vi "Drive Controller.vi"(8 "error in":errorcluster) -> ()   [LabVIEW 2020]
doc: "This VI executes continuously carrying out the current operation and responding to updates or new operation requests. It will often contain the timing or control code that is difficult to place directly in TeleOp. This VI generally opens all sensors and motors and isolates the rest of the robot code from knowing implementation details of how the operations are carried out."
uses:
  <vilib>/Rock Robotics/WPI/ThirdParty/REV Robotics/REVLib/Typedef/Spark MAX Control Type.ctl
  Drive Setpoints.ctl
  Drive Operations.ctl
  swerve/Type Definitions/Data/Robot Velocities.ctl
  <vilib>/Platform/TimedLoop/XDataNode/timing_clust.ctl
  <vilib>/Platform/TimedLoop/XDataNode/nitl_modes.ctl
  <vilib>/Platform/TimedLoop/XDataNode/wakeup.ctl
  <vilib>/Rock Robotics/WPI/ThirdParty/Phoenix-LabVIEW/Motor Controller/Controls/CTRE_Phoenix_MotorControl_ControlMode.ctl
  <vilib>/Rock Robotics/WPI/DriverStation/WPI_DriverStationRobotMode2.ctl
  9a6d1fe9-8481-493e-9338-0d478725c978.vi
  <vilib>/Analysis/_algsub.llb/Real Vector Norm.vi
  <vilib>/Analysis/coordinate.llb/2D Cartesian Coordinate Rotation (Scalar).vi
  Framework/Robot Global Data.vi
  <vilib>/Platform/TimedLoop/XDataNode/XDataNode.xnode
  <vilib>/Analysis/NI_AALPro.lvlib
  <vilib>/Platform/TimedLoop/XDataNode/XDNodeRunTimeDep.lvlib
panel:
  in  "Drive Controller Diagnostics":T1(tab)
  out "Swerve Visualizer":cluster{dbl[], dbl[]}[](graph)
  out "Pod Comparisons (Diff -> Setpoint - Actual)":T2
  out "Robot Pose":cluster{cluster{dbl, dbl}[]}[](graph)
  out "Robot Velocities (ft and deg)/s":cluster{"vx":dbl, "vy":dbl, "w":dbl}
  out "Robot Position (ft)":cluster{"x":dbl, "y":dbl, "theta":dbl}
  in  "Reset Pose":cluster{"vx":dbl, "vy":dbl, "w":dbl}
  in  "Reset?":bool
  out "Speed":dbl
  in  "Reserve Setpoints":T3
  in  "Reserve Control Mode":T4
  in  "Reserve Add Angle Offsets?":bool
  out "Auto Time Delta (ms)":u32(graph)
  out "(Calibration) Steering Angles":T3
  out "Current\nCmd":string
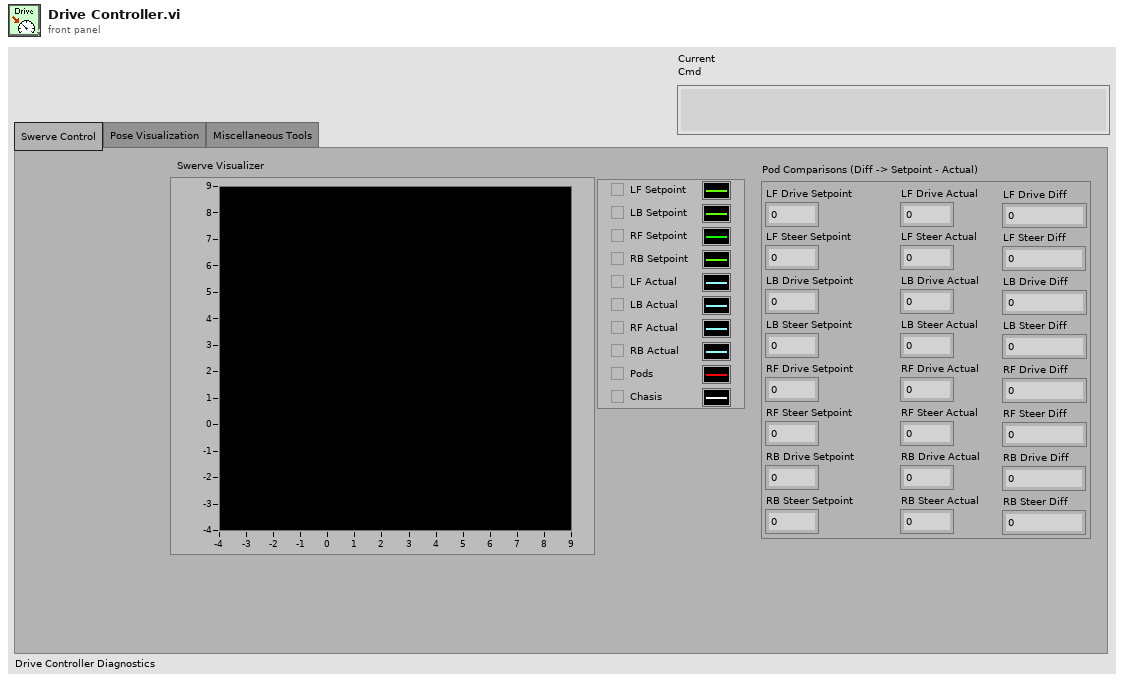
[diagram p1: front panel]
types:
  T1 = enum32{"Swerve Control", "Pose Visualization", "Miscellaneous Tools"}
  T2 = cluster{"LF Drive Setpoint":dbl, "LF Steer Setpoint":dbl, "LB Drive Setpoint":dbl, "LB Steer Setpoint":dbl, "RF Drive Setpoint":dbl, "RF Steer Setpoint":dbl, "RB Drive Setpoint":dbl, "RB Steer Setpoint":dbl, "LF Drive Actual":dbl, "LF Steer Actual":dbl, "LB Drive Actual":dbl, "LB Steer Actual":dbl, "RF Drive Actual":dbl, "RF Steer Actual":dbl, "RB Drive Actual":dbl, "RB Steer Actual":dbl, "LF Drive Diff":dbl, "LF Steer Diff":dbl, "LB Drive Diff":dbl, "LB Steer Diff":dbl, "RF Drive Diff":dbl, "RF Steer Diff":dbl, "RB Drive Diff":dbl, "RB Steer Diff":dbl}
  T3 = cluster{"Left Front":dbl, "Left Back":dbl, "Right Front":dbl, "Right Back":dbl}
  T4 = typedef "Spark MAX Control Type.ctl" = enum16{"Percent VBus", "Voltage", "Velocity", "Position", "Smart Motion", "Current", "Smart Velocity"}
  T5 = cluster{"Time (s)":dbl, "Command out":cluster{"Name":string, "vi reference":refnum<vi>, i32[], variant[]}}
  T6 = typedef "Drive Setpoints.ctl" = cluster{"Operation":T7, "Robot Velocities":T8, "Auto Data":cluster{"Auto Velocities":T8[], "Auto Positions":cluster{"x":dbl, "y":dbl, "th":dbl}[], "Auto Commands":cluster{dbl, "Command out":cluster{"Name":string, "vi reference":refnum<vi>, i32[], variant[]}}[], "Zero Velocity?":bool[]}, "Auto Engage Heading":bool}
  T7 = typedef "Drive Operations.ctl" = enum16{"Reserve", "Read Current", "Immediate", "Calibrate", "Auto", "Auto Engage", "Brake"}
  T8 = typedef "Robot Velocities.ctl" = cluster{"X Velocity":dbl, "Y Velocity":dbl, "Rotational \nVelocity":dbl}
  T9 = typedef "(NEO-NEO-ThroughBore-Pigeon2) Swerve.ctl" = cluster{"Drive Motors (NEO)":T10, "Steer Motors (NEO)":T10, "Pigeon2":T16, "Radii (ft)":T18}
  T10 = typedef "(NEO & NEO 550) 4 Motor Set.ctl" = cluster{"Left Front":T11, "Left Back":T11, "Right Front":T11, "Right Back":T11}
  T11 = typedef "WPI_MotorControlDeviceRef.ctl" = cluster{"DeviceStatus":errorcluster, "Type":T12, "PWM":cluster{"PWM Channel":T13, "DeadBand":T14}, "CAN":cluster{"Device Number":u8, "SetOutput VI Ref":variant, "GetOutput VI Ref":variant, "Enable VI Ref":variant, "Disable VI Ref":variant, "Data":variant}, "Invert":bool, "DIO PWM":cluster{"PWM \"Enable\" Channel":T13, "DIOChannel":T15, "PWM Rate":dbl}}
  T12 = typedef "WPI_MotorControlType.ctl" = enum16{"PWM", "CAN", "DIO PWM"}
  T13 = typedef "FPGA_DIOPWMChannel.ctl" = enum8{"PWM 0", "PWM 1", "PWM 2", "PWM 3", "PWM 4", "PWM 5", "PWM 6", "PWM 7", "PWM 8", "PWM 9", "PWM MXP 0", "PWM MXP 1", "PWM MXP 2", "PWM MXP 3", "PWM MXP 4", "PWM MXP 5", "PWM MXP 6", "PWM MXP 7", "PWM MXP 8", "PWM MXP 9", "Invalid"}
  T14 = typedef "WPI_PWMDeadband.ctl" = cluster{"Name":string, "maxPositivePwm":i32, "minPositivePwm":i32, "centerPwm":i32, "maxNegativePwm":i32, "minNegativePwm":i32, "angularRange":u16}
  T15 = typedef "FPGA_DIOChannel.ctl" = enum8{"DIO 0", "DIO 1", "DIO 2", "DIO 3", "DIO 4", "DIO 5", "DIO 6", "DIO 7", "DIO 8", "DIO 9", "DIO MXP 0", "DIO MXP 1", "DIO MXP 2", "DIO MXP 3", "DIO MXP 4", "DIO MXP 5", "DIO MXP 6", "DIO MXP 7", "DIO MXP 8", "DIO MXP 9", "DIO MXP 10", "DIO MXP 11", "DIO MXP 12", "DIO MXP 13", "DIO MXP 14", "DIO MXP 15", "SPI Port CS1", "SPI Port CS2", "SPI Port CS3", "SPI Port MISO", "SPI Port MOSI", "Invalid"}
  T16 = typedef "CTRE_PigeonIMU_DeviceRef.ctl" = cluster{"DeviceStatus":errorcluster, "Device Number":u8, "Type":T17, "Device ID":u32, "Handle":u64, "UsageFrame":u32, "Library Path":path}
  T17 = typedef "CTRE_PigeonIMU_ConnectionType.ctl" = u32
  T18 = typedef "Pod Positions.ctl" = cluster{"Left Front Position":dbl[], "Left Back Position":dbl[], "Right Front Position":dbl[], "Right Back Position":dbl[]}
  T19 = typedef "Command Status Info.ctl" = cluster{"Name":string, "Status":T20, "notifier out":T21}
  T20 = typedef "Completion Status.ctl" = enum16{"Successful", "Aborted", "Incomplete"}
  T21 = typedef "Completion Notifier.ctl" = refnum<notifier>
  T22 = cluster{"SubSystem Data":T6, cluster{"Start Time (ms)":u32, "Iterations":i32}, cluster{"Command Info":T19, "Description":string, "Default Command":T6, "queue out":refnum<queue>, "Subsystem Name":string}}
  T23 = cluster{"Auto Velocities":T8[], "Auto Positions":cluster{"x":dbl, "y":dbl, "th":dbl}[], "Auto Commands":cluster{dbl, "Command out":cluster{"Name":string, "vi reference":refnum<vi>, i32[], variant[]}}[], "Zero Velocity?":bool[]}
  T24 = cluster{"Field Centric?":bool, "SnapToScore":bool, "TranslationalAlign":bool}
  T25 = typedef "Pod Setpoints.ctl" = cluster{"Left Front":cluster{"Velocity":dbl, "Theta":dbl}, "Left Back":cluster{"Velocity":dbl, "Theta":dbl}, "Right Front":cluster{"Velocity":dbl, "Theta":dbl}, "Right Back":cluster{"Velocity":dbl, "Theta":dbl}}
  T26 = typedef "CTRE_Phoenix_MotorControl_ControlMode.ctl" = u16
  T27 = typedef "Angle State.ctl" = enum16{"Ground", "Close to balanced", "Balanced", "Tilted"}
  T28 = cluster{"SubSystem Data":T6, cluster{"Start Time (ms)":u32, "Iterations":i32}, "Default Command Arguments":cluster{"Command Info":T19, "Description":string, "Default Command":T6, "queue out":refnum<queue>, "Subsystem Name":string}}
  T29 = typedef "XDNodeRunTimeDep.lvlib/timing_clust.ctl" = cluster{"Expected End [f-1]":u64, "Actual End [f-1]":u64, "Finished Late? [f-1]":bool, "Expected End [i-1]":u64, "Actual End [i-1]":u64, "Finished Late? [i-1]":bool, "Expected Start [i]":u64, "Actual Start [i]":u64, "Expected Start [f]":u64, "Actual Start [f]":u64, "Source Name":string, "Structure Name":string, "Period":i64, "Deadline":i64, "Offset":i64, "Start":i64, "Priority":i32, "Timeout":i32, "Mode":T30, "Wakeup Reason":T31, "Error":errorcluster, "Source Type":string, "Secondary Source Type":string, "Global End Time":u64, "Global Start Time":u64, "Frame Duration":u64, "Iteration Duration":u64, "Assigned CPU":i32, "I/O Scan Engine Mode":u32}
  T30 = typedef "XDNodeRunTimeDep.lvlib/nitl_modes.ctl" = enum32{"No Change", "Process missed periods, maintain original phase", "Discard missed periods, maintain original phase", "Process missed periods, ignore original phase", "Discard missed periods, ignore original phase"}
  T31 = typedef "XDNodeRunTimeDep.lvlib/wakeup.ctl" = enum32{"Normal", "Aborted", "Asynchronous wakeup", "Timing source error", "Timed loop error", "Timeout"}
  T32 = typedef "WPI_DriverStationRobotMode2.ctl" = enum16{"Autonomous Disabled", "Autonomous Enabled", "Teleop Disabled", "Teleop Enabled", "Disconnected", "Finish", "Test Disabled", "Test Enabled", "Emergency Stopped"}
  T33 = cluster{dbl, "Command out":cluster{"Name":string, "vi reference":refnum<vi>, i32[], variant[]}}[]
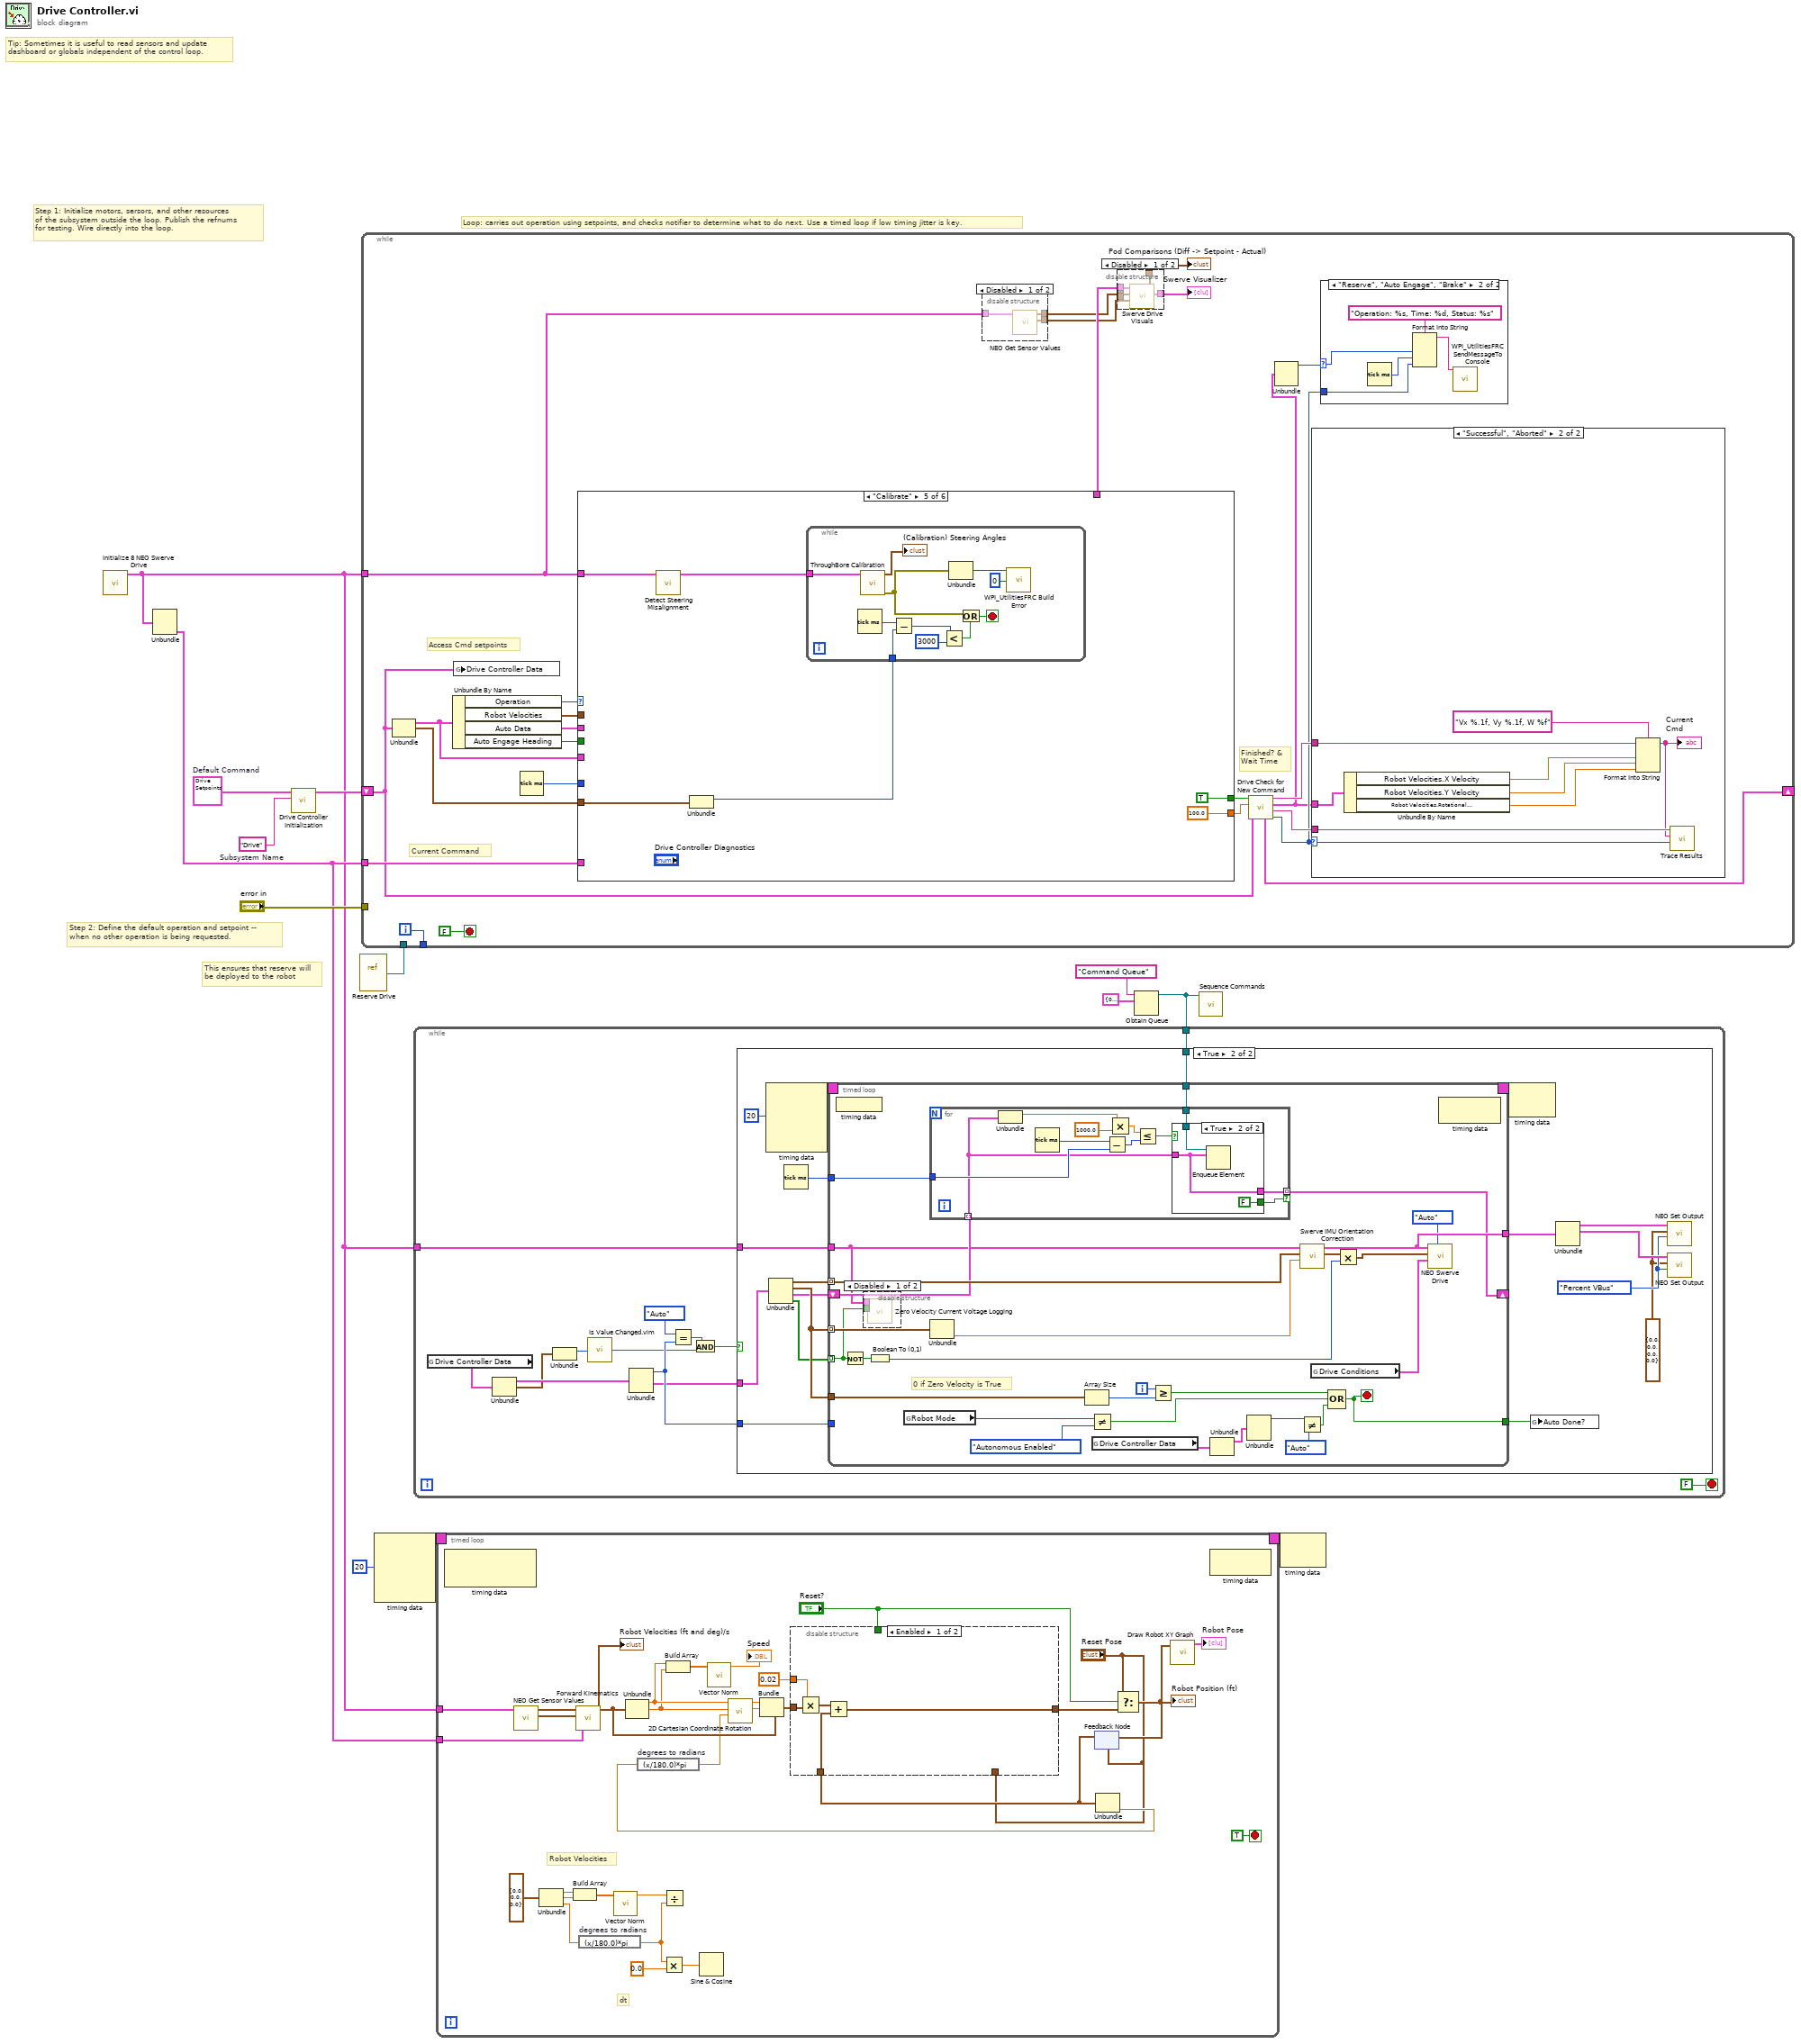
[diagram p0: block diagram]
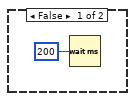
[diagram p2: hidden frame]
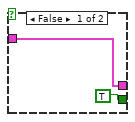
[diagram p4: hidden frame]
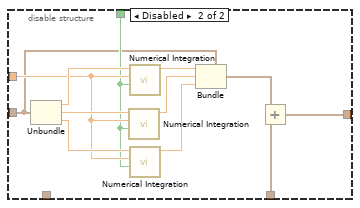
[diagram p5: hidden frame]
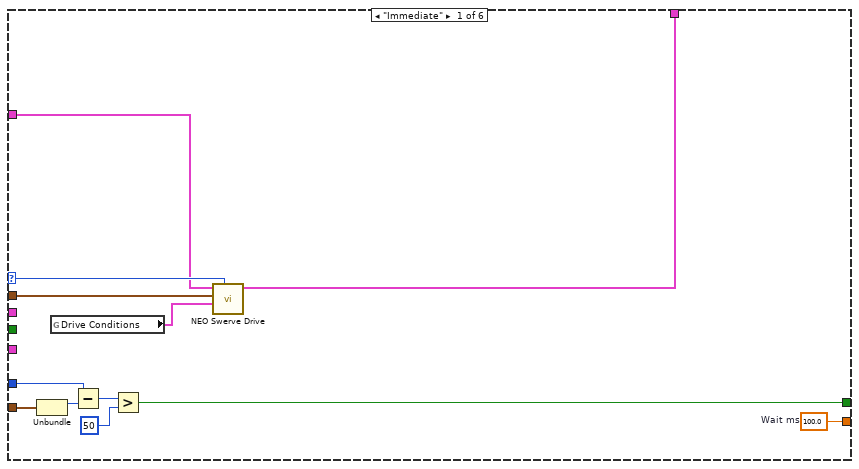
[diagram p9: hidden frame]
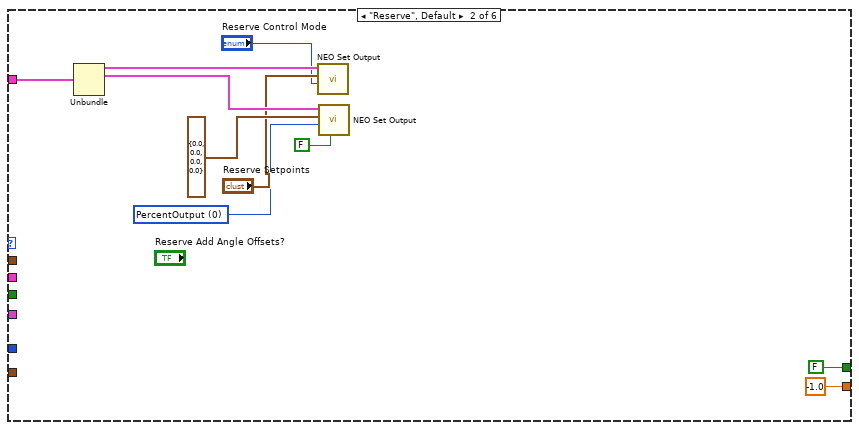
[diagram p10: hidden frame]
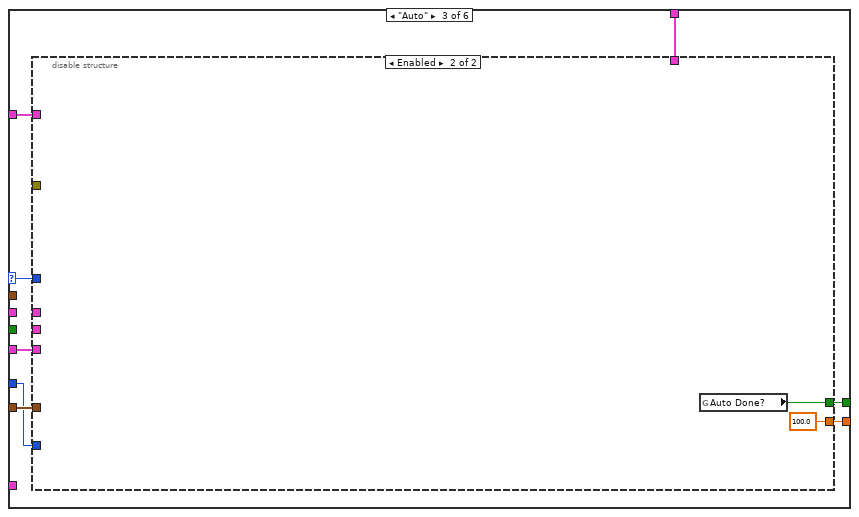
[diagram p11: hidden frame]
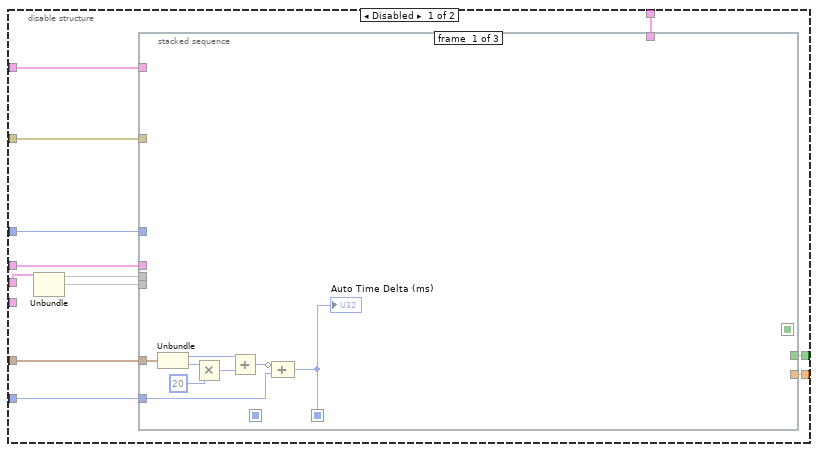
[diagram p12: hidden frame]
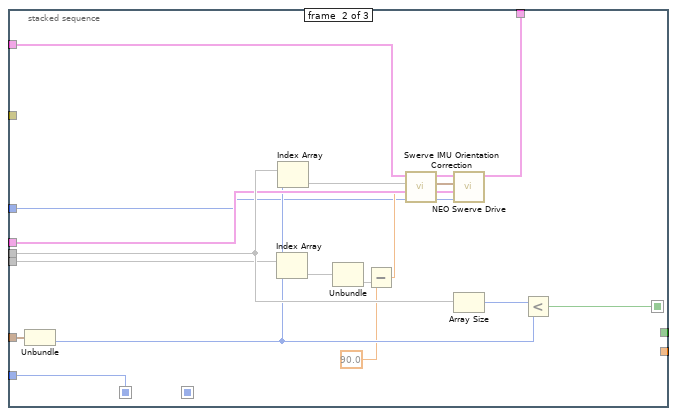
[diagram p13: hidden frame]
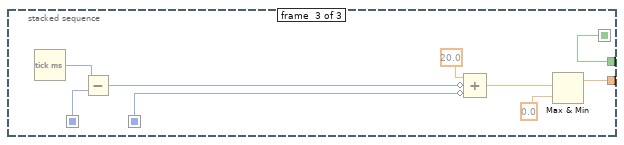
[diagram p14: hidden frame]
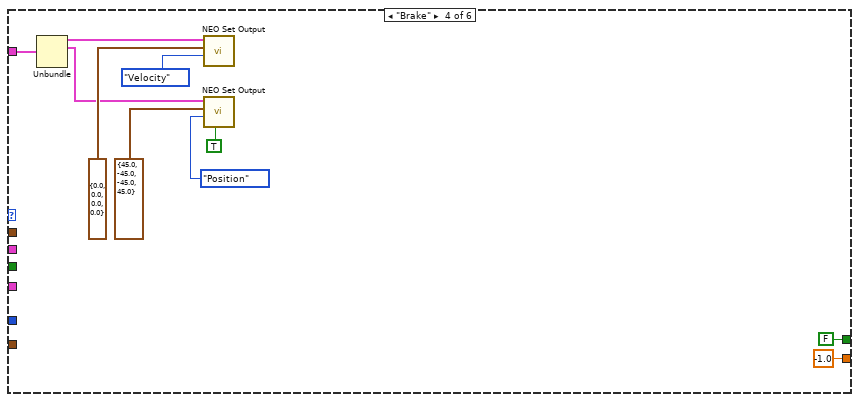
[diagram p15: hidden frame]
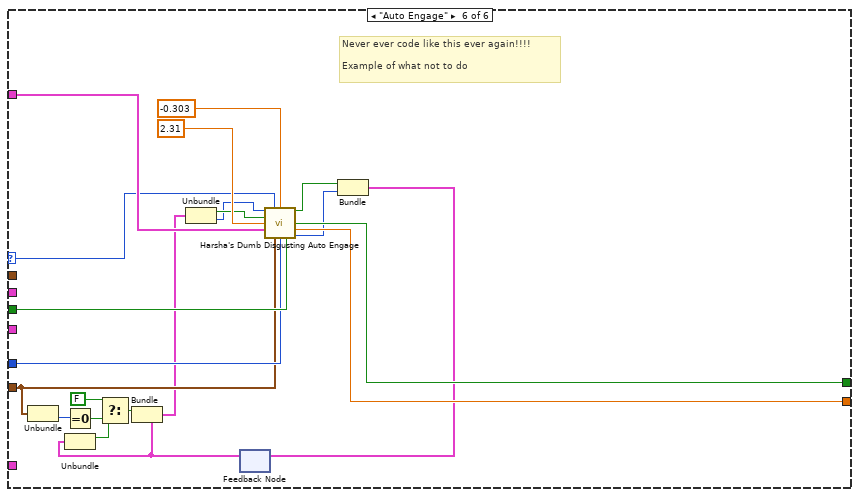
[diagram p16: hidden frame]
diagram:
  w9 = T6 {"Operation"=enum."Reserve", "Robot Velocities"={"X Velocity"=0.0, "Y Velocity"=0.0, "Rotational \nVelocity"=0.0}, "Auto Data"={"Auto Velocities"=[], "Auto Positions"=[], "Auto Commands"=[], "Zero Velocity?"=[]}, "Auto Engage Heading"=FALSE}  # Default Command
  w13 = "Drive"  # Subsystem Name
  # "This ensures that reserve will\nbe deployed to the robot"
  # "Step 2: Define the default operation and setpoint --\nwhen no other operation is being requested."
  # "Step 1: Initialize motors, sersors, and other resources\nof the subsystem outside the loop. Publish the refnums\nfor testing. Wire directly into the loop."
  # "Loop: carries out operation using setpoints, and checks notifier to determine what to do next. Use a timed loop if low timing jitter is key."
  # "Tip: Sometimes it is useful to read sensors and update\ndashboard or globals independent of the control loop."
  n1 = call "Initialize 8 NEO Swerve Drive.vi"() -> ("Motors"=w4:T9)  [unwired: 10 in, 1 out]
  n2 = Unbundle(w4) -> ("Radii (ft)"=w8:T18)  [unwired: 3 out]
  n3 = call "Drive Controller Initialization.vi"("Subsystem Name"=w13, "Default Command"=w9) -> ("Current Command"=w11:T22)  [unwired: 9 in]
  n4 = vi-ref "Reserve Drive.vi"() -> (w10:refnum<vi>)
  n5 = while {
    shift-right: [w28] -> _
    shift-left: w11 -> [w14]
    tunnel: [w37] -> _
    tunnel: "error in" -> [_]
    tunnel: w10 -> [_]
    tunnel: w4 -> [w24]
    tunnel: w8 -> [w31]
    i -> [w37]
    stop <- FALSE stop-if-true
    # "Current Command"
    # "Access Cmd setpoints"
    # "Finished? &\nWait Time"
    n6 = Unbundle(w14) -> ("SubSystem Data"=w17:T6, w15:cluster{"Start Time (ms)":u32, "Iterations":i32})  [unwired: 1 out]
    n7 = Unbundle By Name(w17) -> ("Operation"=w21:T7, "Robot Velocities"=w32:T8, "Auto Data"=w23:T23, "Auto Engage Heading"=w22:bool)
    n8 = global write "Robot Global Data.vi" "Drive Controller Data"(w14) -> ()
    n9 = Tick Count (ms)() -> (millisecond timer value=w16:u32)
    n10 = case shown="\"Calibrate\"" w21 {
      selector: w21 -> [w55 _ w75 _ _ w175]
      tunnel: [w63 -1.0 ("Infinite") w77 -1.0 ("Infinite") 100.0 ("Infinite") w171] -> w36
      tunnel: [w58 FALSE ("ignore previous (F)") w79 FALSE ("Boolean out") TRUE ("ignore previous (F)") w172] -> w35
      tunnel: w15 -> [w62 _ w81 _ w144 w167]
      tunnel: w16 -> [w57 _ w76 _ _ w173]
      tunnel: w32 -> [w52 _ _ _ _ _]
      tunnel: w24 -> [w53 w71 w80 w140 w142 w178]
      tunnel: w31 -> [_ _ _ _ _ _]
      tunnel: [w56 _ w78 _ _ _] -> w27
      tunnel: w17 -> [_ _ w74 _ _ _]
      tunnel: w23 -> [_ _ _ _ _ _]
      tunnel: w22 -> [_ _ _ _ _ w174]
      frame "Immediate" {
        w63 = 100.0  # Wait ms
        n11 = Unbundle(w62) -> ("Start Time (ms)"=w61:u32)  [unwired: 1 out]
        n12 = global read "Robot Global Data.vi" "Drive Conditions"() -> (w54:T24)
        n13 = Subtract(x=w57, y=w61) -> (x-y=w60:u32)
        n14 = Greater?(x=w60, y=u32 50) -> (0:w58:bool)
        n15 = call "NEO Swerve Drive.vi"("Operation"=w55, "Drive Conditions"=w54, "Robot Velocities"=w52, "Swerve Drive"=w53) -> ("Pod Setpoints (ft/s and deg)"=w56:T25)  [unwired: 7 in]
      }
      frame "Reserve", Default {
        w65 = T26 0 items=["PercentOutput"=0, "Position"=1, "Velocity"=2, "Current"=3, "Follower"=5, "MotionProfile"=6, "MotionMagic"=7, "MotionProfileArc"=10, "Disabled"=15] ("Control Mode")
        n16 = Unbundle(w71) -> ("Drive Motors (NEO)"=w70:T10, "Steer Motors (NEO)"=w69:T10)  [unwired: 2 out]
        n17 = call "NEO Set Output.vi"("Control Mode"="Reserve Control Mode", "Setpoints"="Reserve Setpoints", "Motors"=w70) -> ()  [unwired: 9 in]
        n18 = call "NEO Set Output.vi"("Add Angle Offsets?"=FALSE, "Control Mode"=w65, "Setpoints"=T3 {"Left Front"=0.0, "Left Back"=0.0, "Right Front"=0.0, "Right Back"=0.0}, "Motors"=w69) -> ()  [unwired: 8 in]
      }
      frame "Auto" {
        n19 = disable-structure shown="Enabled" {
          disable-tunnel: w81 -> [w93 _]
          disable-tunnel: w80 -> [w92 _]
          disable-tunnel: [w91 w129] -> w79
          disable-tunnel: [w90 _] -> w78
          disable-tunnel: [w89 100.0] -> w77
          disable-tunnel: w76 -> [w88 _]
          disable-tunnel: _ -> [w87 _]
          disable-tunnel: _ -> [w86 _]
          disable-tunnel: _ -> [w85 _]
          disable-tunnel: w75 -> [w82 _]
          disable-tunnel: w74 -> [_ _]
          frame Disabled {
            n20 = Unbundle(w85) -> ("Auto Velocities"=w84, "Auto Positions"=w83)  [unwired: 1 out]
            n21 = stacked-sequence {
              seq-local: [_ w116 _] -> [_ _ w128]
              seq-local: [_ w115 _] -> [_ _ w123]
              seq-local: [w94 _ _] -> [_ _ w120]
              tunnel: w93 -> [w101 w118 _]
              tunnel: w84 -> [_ w117 _]
              tunnel: w92 -> [_ w112 _]
              tunnel: [_ w114 _] -> w90
              tunnel: w88 -> [w95 w115 _]
              tunnel: w87 -> [_ _ _]
              tunnel: [_ _ w128] -> w91
              tunnel: [_ _ w124] -> w89
              tunnel: w86 -> [_ w111 _]
              tunnel: w83 -> [_ w110 _]
              tunnel: w82 -> [_ w102 _]
              frame #0 {
                n22 = Unbundle(w101) -> ("Start Time (ms)"=w98:u32, "Iterations"=w100:i32)
                n23 = Multiply(x=w100, y=20) -> (x*y=w97:i32)
                n24 = Add(x=w98, y=w97) -> (x+y=w96:u32)
                n25 = Compound Arithmetic op=ADD(invert w96, w95) -> (w94:u32)
                "Auto Time Delta (ms)" <- w94
              }
              frame #1 {
                n26 = Unbundle(w118) -> ("Iterations"=w109:i32)  [unwired: 1 out]
                n27 = Index Array(array=w110, index=w109) -> (element=w108)
                n28 = Index Array(array=w117, index=w109) -> (element=w113)
                n29 = Unbundle(w108) -> (w107)  [unwired: 2 out]
                n30 = Subtract(x=90.0 ("y"), y=w107) -> (x-y=w105:dbl)
                n31 = call "Swerve IMU Orientation Correction.vi"("Setpoint"=w105, "Robot Velocities In"=w113, "Motors In"=w112) -> ("Robot Velocities Out"=w104:T8, "Motors Out"=w103:T9)  [unwired: 7 in]
                n32 = call "NEO Swerve Drive.vi"(8:w102, "Drive Conditions"=w111, "Robot Velocities"=w104, "Swerve Drive"=w103) -> ("Pod Setpoints (ft/s and deg)"=w114:T25)  [unwired: 7 in]
                n33 = Array Size(array=w117) -> (size(s)=w119:i32)
                n34 = Less?(x=w119, y=w109) -> (x < y?=w116:bool)
              }
              frame #2 {
                n35 = Tick Count (ms)() -> (millisecond timer value=w121:u32)
                n36 = Subtract(x=w121, y=w123) -> (x-y=w122:u32)
                n37 = Compound Arithmetic op=unknown(20.0 ("Infinite"), invert w122, invert w120) -> (w126:dbl)
                n38 = Max & Min(x=w126, y=0.0) -> (max(x,y)=w124:dbl)  [unwired: 1 out]
              }
            }
          }
          frame Enabled {
            n39 = global read "Robot Global Data.vi" "Auto Done?"() -> (w129:bool)
          }
        }
      }
      frame "Brake" {
        n40 = Unbundle(w140) -> ("Drive Motors (NEO)"=w139:T10, "Steer Motors (NEO)"=w137:T10)  [unwired: 2 out]
        n41 = call "NEO Set Output.vi"("Control Mode"=Spark_MAX_Control_Type."Velocity", "Setpoints"=T3 {"Left Front"=0.0, "Left Back"=0.0, "Right Front"=0.0, "Right Back"=0.0}, "Motors"=w139) -> ()  [unwired: 9 in]
        n42 = call "NEO Set Output.vi"("Add Angle Offsets?"=TRUE, "Control Mode"=Spark_MAX_Control_Type."Position", "Setpoints"=T3 {"Left Front"=45.0, "Left Back"=-45.0, "Right Front"=-45.0, "Right Back"=45.0}, "Motors"=w137) -> ()  [unwired: 8 in]
      }
      frame "Calibrate" {
        n43 = call "Detect Steering Misalignment.vi"("Motors In"=w142) -> ("Motors Out"=w141:T9)  [unwired: 10 in]
        n44 = Unbundle(w144) -> ("Start Time (ms)"=w143:u32)  [unwired: 1 out]
        n45 = while {
          tunnel: w141 -> [w151]
          tunnel: w143 -> [w156]
          stop <- w157 stop-if-true
          n46 = Tick Count (ms)() -> (millisecond timer value=w155:u32)
          n47 = call "ThroughBore Calibration.vi"("Motors"=w151) -> ("error out"=w148:errorcluster, "Steering Angles"=→"(Calibration) Steering Angles":cluster{"LF":dbl, "LB":dbl, "RF":dbl, "RB":dbl})  [unwired: 9 in]
          n48 = Subtract(x=w155, y=w156) -> (x-y=w154:u32)
          n49 = Less?(x=w154, y=u32 3000) -> (x < y?=w152:bool)
          n50 = Unbundle(w148) -> ("code"=w147:i32)  [unwired: 2 out]
          n51 = Or(x=w148, y=w152) -> (x .or. y?=w157:bool)
          n52 = call <vilib>:"WPI_UtilitiesFRC Build Error.vi"("error code"=w147, "chain levels to remove (1)"=0) -> ()  [unwired: 3 in, 11 out]
        }
      }
      frame "Auto Engage" {
        # "Never ever code like this ever again!!!!\n\nExample of what not to do"
        n53 = Unbundle(w167) -> ("Iterations"=w166:i32)  [unwired: 1 out]
        n54 = Equal To 0?(x=w166) -> (x = 0?=w165:bool)
        n55 = feedback #1() -> (w164:cluster{"Boolean 3":bool, "New State":T27})  [unwired: 1 in]
        n56 = Unbundle(w164) -> ("Boolean 3"=w163:bool)  [unwired: 1 out]
        n57 = Select(t=FALSE, s=w165, f=w163) -> (s? t:f=w161:bool)
        n58 = Bundle(cluster=w164, "Boolean 3"=w161) -> (w160:cluster{"Boolean 3":bool, "New State":T27})  [unwired: 1 in]
        n59 = Unbundle(w160) -> ("Boolean 3"=w159:bool, "New State"=w158:T27)
        n60 = call "Harsha's Dumb Disgusting Auto Engage.vi"("State"=w158, "Operation"=w175, "Roll"=-0.303, "Boolean in"=w159, "Pitch"=2.31, "Motors"=w178, "Cluster"=w167, "millisecond timer value"=w173, "Heading"=w174) -> ("Boolean 3"=w170:bool, "Boolean out"=w172:bool, "Infinite"=w171:dbl, "New State"=w169:T27)  [unwired: 1 in, 2 out]
        n61 = Bundle("Boolean 3"=w170, "New State"=w169) -> (w168:cluster{"Boolean 3":bool, "New State":T27})  [unwired: 1 in]
        n62 = feedback-in #1(w168) -> ()
      }
    }
    n63 = disable-structure shown="Disabled" {
      disable-tunnel: w24 -> [w46 _]
      disable-tunnel: [w45 _] -> w26
      disable-tunnel: [w44 _] -> w25
      frame Disabled {
        n64 = call "NEO Get Sensor Values.vi"("Swerve Motors"=w46) -> ("Steer Angles (degrees)"=w44:T3, "Drive Velocities (ft/s)"=w45:T3)  [unwired: 9 in]
      }
      frame Enabled {
      }
    }
    n65 = disable-structure shown="Disabled" {
      disable-tunnel: [w51 _] -> w30
      disable-tunnel: [w50 _] -> w29
      disable-tunnel: w27 -> [w49 _]
      disable-tunnel: w26 -> [w48 _]
      disable-tunnel: w25 -> [w47 _]
      frame Disabled {
        n66 = call "Swerve Drive Visuals.vi"("Steer Angles (degrees)"=w47, "Drive Velocities (ft/s)"=w48, "Pod Setpoints (ft/s and deg)"=w49) -> ("Swerve Visualizer"=w50:cluster{dbl[], dbl[]}[], "Pod Comparisons (Diff -> Setpoint - Actual)"=w51:T2)  [unwired: 7 in]
      }
      frame Enabled {
      }
    }
    "Pod Comparisons (Diff -> Setpoint - Actual)" <- w30
    "Swerve Visualizer" <- w29
    n67 = call "Drive Check for New Command.vi"("input cluster"=w14, "Wait time (ms)"=w36, "Finished?"=w35) -> ("Completion"=w20:T20, "Subsystem Name"=w33:string, "Current Command"=w19:T6, "Initial Trace String"=w34:string, "Next Command"=w28:T28)  [unwired: 4 in]
    n68 = Unbundle(w19) -> ("Operation"=w18:T7)  [unwired: 3 out]
    n69 = case shown="\"Successful\", \"Aborted\"" w20 {
      selector: w20 -> [_ w179]
      tunnel: w34 -> [_ w186]
      tunnel: w19 -> [_ w187]
      tunnel: w33 -> [_ w185]
      frame "Incomplete", Default {
        # "Continuing current command"
      }
      frame "Successful", "Aborted" {
        # "Report and setup for next command"
        n70 = Unbundle By Name(w187) -> ("Robot Velocities.X Velocity"=w183:dbl, "Robot Velocities.Y Velocity"=w184:dbl, "Robot Velocities.Rotational \nVelocity"=w180:dbl)
        n71 = Format Into String(format string="Vx %.1f, Vy %.1f, W %f", initial string=w186, w183, w184, w180) -> (resulting string=w181:string)  [unwired: 1 in, 1 out]
        "Current\nCmd" <- w181
        n72 = call <vilib>:"Trace Results.vi"("Status of previous command"=w179, "Description"=w181, "Subsystem"=w185) -> ()  [unwired: 9 in]
      }
    }
    n73 = case shown="\"Reserve\", \"Auto Engage\", \"Brake\"" w18 {
      selector: w18 -> [_ w39]
      tunnel: w20 -> [_ w40]
      frame Default {
      }
      frame "Reserve", "Auto Engage", "Brake" {
        n74 = Tick Count (ms)() -> (millisecond timer value=w42:u32)
        n75 = Format Into String(format string="Operation: %s, Time: %d, Status: %s", w39, w42, w40) -> (resulting string=w41:string)  [unwired: 2 in, 1 out]
        n76 = call <vilib>:"WPI_UtilitiesFRC SendMessageToConsole.vi"("Message"=w41) -> ()  [unwired: 14 in, 1 out]
      }
    }
  }
  n77 = node-c288(i64 20 ("Period")) -> (w7:T29)  [unwired: 3 in]
  n78 = timed-loop {
    tunnel: w4 -> [w218]
    tunnel: w8 -> [w216]
    timing: w7 -> [_]
    timing-out: [_] -> w6
    stop <- TRUE stop-if-true
    # "Robot Velocities"
    # "dt"
    n79 = node-c288() -> ()  [unwired: 1 in, 2 out]
    n80 = call "NEO Get Sensor Values.vi"("Swerve Motors"=w218) -> ("Steer Angles (degrees)"=w209:T3, "Drive Velocities (ft/s)"=w210:T3)  [unwired: 9 in]
    n81 = Unbundle(T8 {"X Velocity"=0.0, "Y Velocity"=0.0, "Rotational \nVelocity"=0.0} ("Robot Velocities (ft and deg)/s")) -> ("X Velocity"=w193:dbl, "Y Velocity"=w194:dbl, "Rotational \nVelocity"=w198:dbl)
    n82 = Build Array(w193, w194) -> (w195:dbl[])
    n83 = call "Forward Kinematics.vi"("Radii (ft)"=w216, "Steer Angles (degrees)"=w209, "Drive Velocities (ft/s)"=w210) -> ("Robot Velocities (ft and deg)/s"=w214:T8)  [unwired: 8 in]
    "Robot Velocities (ft and deg)/s" <- w214
    n84 = expression code="(x/180.0)*pi" "degrees to radians"(w198) -> (w199:dbl)
    n85 = call-poly <vilib>:"Vector Norm.vi"("Input Vector"=w195) -> ("norm"=w196:dbl)  [unwired: 9 in, 1 out]
    n86 = Unbundle(w214) -> ("X Velocity"=w191:dbl, "Y Velocity"=w190:dbl)  [unwired: 1 out]
    n87 = Multiply(x=w199, y=0.0) -> (x*y=w200:dbl)
    n88 = Divide(x=w196, y=w199) -> ()  [unwired: 1 out]
    n89 = Build Array(w191, w190) -> (w189:dbl[])
    n90 = Sine & Cosine(0:w200) -> ()  [unwired: 2 out]
    n91 = call-poly <vilib>:"Vector Norm.vi"("Input Vector"=w189) -> ("norm"=→"Speed":dbl)  [unwired: 9 in, 1 out]
    n92 = feedback #2("Reset Pose") -> (w208:T8)
    n93 = Unbundle(w208) -> ("Rotational \nVelocity"=w203:dbl)  [unwired: 2 out]
    n94 = expression code="(x/180.0)*pi" "degrees to radians"(w203) -> (w206:dbl)
    n95 = call-poly <vilib>:"2D Cartesian Coordinate Rotation.vi"("theta"=w206, "y"=w190, "x"=w191) -> ("y out"=w212:dbl, "x out"=w213:dbl)  [unwired: 6 in, 1 out]
    n96 = Bundle(cluster=w214, "X Velocity"=w213, "Y Velocity"=w212) -> (w211:T8)  [unwired: 1 in]
    n97 = disable-structure shown="Enabled" {
      disable-tunnel: [w223 w225] -> w215
      disable-tunnel: w211 -> [w222 w229]
      disable-tunnel: w208 -> [w221 _]
      disable-tunnel: 0.02 -> [w220 w232]
      disable-tunnel: "Reset?" -> [_ w231]
      disable-tunnel: "Reset Pose" -> [_ w224]
      frame Enabled {
        n98 = Multiply(x=w220, y=w222) -> (x*y=w219:T8)
        n99 = Add(x=w219, y=w221) -> (x+y=w223:T8)
      }
      frame Disabled {
        n100 = Unbundle(w229) -> ("X Velocity"=w235:dbl, "Y Velocity"=w234:dbl, "Rotational \nVelocity"=w233:dbl)
        n101 = call "Numerical Integration.vi"("Reset?"=w231, "dt"=w232, "Data"=w234) -> ("Integrated Data"=w228:dbl)  [unwired: 8 in]
        n102 = call "Numerical Integration.vi"("Reset?"=w231, "dt"=w232, "Data"=w235) -> ("Integrated Data"=w230:dbl)  [unwired: 8 in]
        n103 = call "Numerical Integration.vi"("Reset?"=w231, "dt"=w232, "Data"=w233) -> ("Integrated Data"=w227:dbl)  [unwired: 8 in]
        n104 = Bundle(cluster=w229, "X Velocity"=w230, "Y Velocity"=w228, "Rotational \nVelocity"=w227) -> (w226:T8)
        n105 = Add(x=w226, y=w224) -> (x+y=w225:T8)
      }
    }
    n106 = Select(t="Reset Pose", s="Reset?", f=w215) -> (s? t:f=w204:T8)
    "Robot Position (ft)" <- w204
    n107 = feedback-in #2(w204) -> ()
    n108 = call "Draw Robot XY Graph.vi"("Pose"=w204) -> ("Robot Pose"=→"Robot Pose":cluster{cluster{dbl, dbl}[]}[])  [unwired: 10 in]
    n109 = node-c288() -> ()  [unwired: 1 in, 1 out]
  }
  n110 = Obtain Queue(name (unnamed)="Command Queue", element data type=T5 {"Time (s)"=0.0, "Command out"={"Name"="", "vi reference"=refnum, [], []}} ("element")) -> (queue out=w1:refnum<queue>)  [unwired: 3 in, 2 out]
  n111 = while {
    tunnel: w4 -> [w248]
    tunnel: w1 -> [w241]
    stop <- FALSE stop-if-true
    n112 = global read "Robot Global Data.vi" "Drive Controller Data"() -> (w245:T22)
    n113 = Unbundle(w245) -> ("SubSystem Data"=w247:T6, w240:cluster{"Start Time (ms)":u32, "Iterations":i32})  [unwired: 1 out]
    n114 = Unbundle(w240) -> ("Start Time (ms)"=w239:u32)  [unwired: 1 out]
    n115 = call "Is Value Changed.vim"("value"=w239) -> ("changed or first call?"=w238:bool)
    n116 = Unbundle(w247) -> ("Operation"=w243:T7, "Auto Data"=w242:T23)  [unwired: 2 out]
    n117 = Equal?(x=Drive_Operations."Auto", y=w243) -> (x = y?=w246:bool)
    n118 = And(x=w246, y=w238) -> (x .and. y?=w244:bool)
    n119 = case shown="True" w244 {
      tunnel: w242 -> [_ w260]
      tunnel: w248 -> [_ w266]
      tunnel: w243 -> [_ w261]
      tunnel: w241 -> [_ w256]
      frame False {
        n120 = Wait (ms)(milliseconds to wait=u32 200) -> ()  [unwired: 1 out]
      }
      frame True {
        w263 = Spark_MAX_Control_Type."Percent VBus" ("Control Mode")
        w262 = T3 {"Left Front"=0.0, "Left Back"=0.0, "Right Front"=0.0, "Right Back"=0.0} ("Setpoints")
        n121 = node-c288(i64 20 ("Period")) -> (w269:T29)  [unwired: 3 in]
        n122 = Unbundle(w260) -> ("Auto Velocities"=w259:T8[], "Auto Positions"=w258:cluster{"x":dbl, "y":dbl, "th":dbl}[], "Auto Commands"=w255:T33, "Zero Velocity?"=w253:bool[])
        n123 = Tick Count (ms)() -> (millisecond timer value=w257:u32)
        n124 = timed-loop {
          timing: w269 -> [_]
          timing-out: [_] -> w268
          tunnel: w266 -> [w270]
          tunnel: [w296] -> w254
          tunnel: w261 -> [_]
          tunnel: w259 -> [w295] mode=indexing
          tunnel: w258 -> [w294] mode=indexing
          tunnel: w258 -> [w293]
          tunnel: w257 -> [w292]
          tunnel: w256 -> [w290]
          shift-right: [w287] -> _
          shift-left: w255 -> [w286]
          tunnel: w253 -> [w271] mode=indexing
          tunnel: [w277] -> w252
          i -> [w297]
          stop <- w277 stop-if-true
          # "0 if Zero Velocity is True"
          n125 = node-c288() -> ()  [unwired: 1 in]
          n126 = Not(x=w271) -> (.not. x?=w283:bool)
          n127 = disable-structure shown="Disabled" {
            disable-tunnel: w271 -> [w300 _]
            disable-tunnel: w270 -> [w299 _]
            frame Disabled {
              n128 = call "Zero Velocity Current Voltage Logging.vi"("Zero Velocity?"=w300, "Motors In"=w299) -> ()  [unwired: 10 in]
            }
            frame Enabled {
            }
          }
          n129 = Boolean To (0,1)(Boolean=w283) -> (0, 1=w281:i16)
          n130 = global read "Robot Global Data.vi" "Robot Mode"() -> (w285:T32)
          n131 = for {
            tunnel: w292 -> [w310]
            tunnel: w290 -> [w304]
            tunnel: w286 -> [w303] mode=indexing
            tunnel: [w302] -> w287 mode=indexing if=w301
            n132 = Unbundle(w303) -> (w309:dbl)  [unwired: 1 out]
            n133 = Tick Count (ms)() -> (millisecond timer value=w311:u32)
            n134 = Subtract(x=w311, y=w310) -> (x-y=w306:u32)
            n135 = Multiply(x=w309, y=1000.0) -> (x*y=w307:dbl)
            n136 = Less Or Equal?(x=w307, y=w306) -> (x <= y?=w305:bool)
            n137 = case shown="True" w305 {
              tunnel: w304 -> [_ w316]
              tunnel: w303 -> [w312 w315]
              tunnel: [w312 w315] -> w302
              tunnel: [TRUE FALSE] -> w301
              frame False {
              }
              frame True {
                n138 = Enqueue Element(queue=w316, element=w315) -> ()  [unwired: 2 in, 3 out]
              }
            }
          }
          n139 = Unbundle(w294) -> ("th"=w279:dbl)  [unwired: 2 out]
          n140 = Array Size(array=w293) -> (size(s)=w298:i32)
          n141 = Not Equal?(x=w285, y=WPI_DriverStationRobotMode2."Autonomous Enabled") -> (x != y?=w278:bool)
          n142 = global read "Robot Global Data.vi" "Drive Controller Data"() -> (w276:T22)
          n143 = Greater Or Equal?(x=w297, y=w298) -> (x >= y?=w291:bool)
          n144 = Unbundle(w276) -> ("SubSystem Data"=w275:T6)  [unwired: 2 out]
          n145 = Unbundle(w275) -> ("Operation"=w273:T7)  [unwired: 3 out]
          n146 = call "Swerve IMU Orientation Correction.vi"("Setpoint"=w279, "Robot Velocities In"=w295, "Motors In"=w270) -> ("Robot Velocities Out"=w282:T8, "Motors Out"=w296:T9)  [unwired: 7 in]
          n147 = Not Equal?(x=w273, y=Drive_Operations."Auto") -> (x != y?=w274:bool)
          n148 = global read "Robot Global Data.vi" "Drive Conditions"() -> (w288:T24)
          n149 = Compound Arithmetic op=OR(w291, w278, w274) -> (w277:bool)
          n150 = Multiply(x=w282, y=w281) -> (x*y=w280:T8)
          n151 = call "NEO Swerve Drive.vi"("Operation"=Drive_Operations."Auto", "Drive Conditions"=w288, "Robot Velocities"=w280, "Swerve Drive"=w296) -> ()  [unwired: 7 in, 1 out]
          n152 = node-c288() -> ()  [unwired: 1 in, 1 out]
        }
        n153 = node-c288(w268) -> ()  [unwired: 1 out]
        n154 = global write "Robot Global Data.vi" "Auto Done?"(w252) -> ()
        n155 = Unbundle(w254) -> ("Drive Motors (NEO)"=w265:T10, "Steer Motors (NEO)"=w264:T10)  [unwired: 2 out]
        n156 = call "NEO Set Output.vi"("Control Mode"=w263, "Setpoints"=w262, "Motors"=w265) -> ()  [unwired: 9 in]
        n157 = call "NEO Set Output.vi"("Control Mode"=w263, "Setpoints"=w262, "Motors"=w264) -> ()  [unwired: 9 in]
      }
    }
  }
  n158 = call "Sequence Commands.vi"("queue in"=w1) -> ()  [unwired: 11 in]
  n159 = node-c288(w6) -> ()  [unwired: 1 out]
